vi "Unregister.vi"(8 "Error In":errorcluster, 9 "Registrant Enq":refnum<class "Message Enqueuer.lvclass">, 11 "Event Source In":refnum<class "Event Source.lvclass">) -> (0 "Error Out":errorcluster, 3 "Event Source Out":refnum<class "Event Source.lvclass">)   [LabVIEW 2019, in "Event Source.lvlib" / "Event Source.lvclass"]
doc: "This method unregisters a specific Actors Enqueuer from all Events he is listening to from this Event Source Actor."
uses:
  Event Source.lvclass
  <resource>/AFDebug/AF Debug.lvlib
  <vilib>/ActorFramework/Message Enqueuer/Message Enqueuer.lvclass
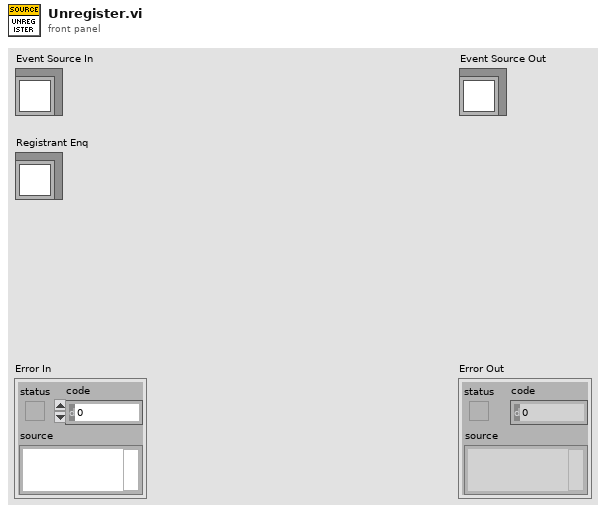
[diagram p1: front panel]
types:
  T1 = map{string, map{refnum<class "Message Enqueuer.lvclass">, refnum<class "Event Generated Msg.lvclass">}}
  T2 = map{refnum<class "Message Enqueuer.lvclass">, refnum<class "Event Generated Msg.lvclass">}
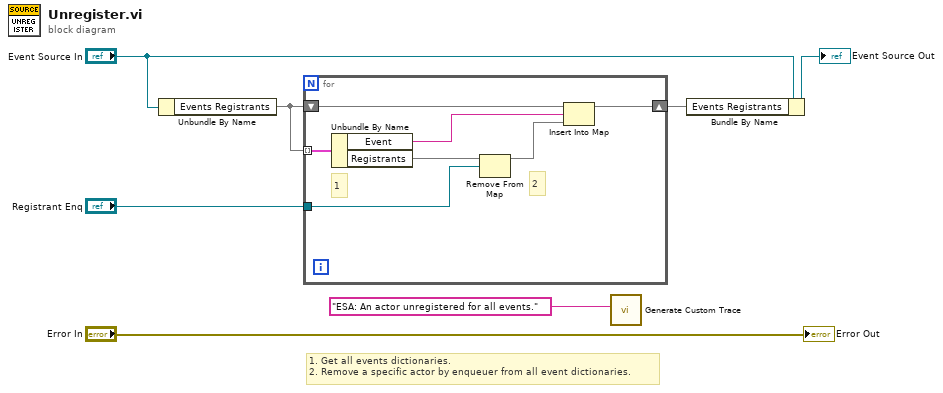
[diagram p0: block diagram]
diagram:
  # "1. Get all events dictionaries.\n2. Remove a specific actor by enqueuer from all event dictionaries."
  n1 = Unbundle By Name("Event Source In") -> ("Events Registrants"=w5:T1)
  n2 = for {
    tunnel: w5 -> [w12] mode=indexing
    tunnel: "Registrant Enq" -> [w13]
    shift-right: [w8] -> w3
    shift-left: w5 -> [w11]
    # "2"
    # "1"
    n3 = Unbundle By Name(w12) -> ("Event"=w10:string, "Registrants"=w14:T2)
    n4 = Remove From Map(10:w13, 11:w14) -> (3:w9:T2)  [unwired: 2 out]
    n5 = Insert Into Map(map in=w11, key=w10, value=w9) -> (map out=w8:T1)  [unwired: 2 out]
  }
  n6 = call <resource>:"Generate Custom Trace.vi"("Custom Action"="ESA: An actor unregistered for all events.") -> ()  [unwired: 11 in]
  n7 = Bundle By Name(cluster="Event Source In", "Events Registrants"=w3) -> (→"Event Source Out":refnum<class "Event Source.lvclass">)
  "Error Out" <- "Error In"
